vi "Taskbar Cleanup.vi"(4 "error in (no error)":errorcluster, 5 "hIcon":i32, 6 "hWnd":T1, 7 "siwutil32":T2) -> (0 "error out":errorcluster)   [LabVIEW 2011]
uses:
  Summitek EXT/Win32/SIWUTIL32/siwutil32.ctl
  Summitek EXT/Win32/WinUSER/Windows/hWnd.ctl
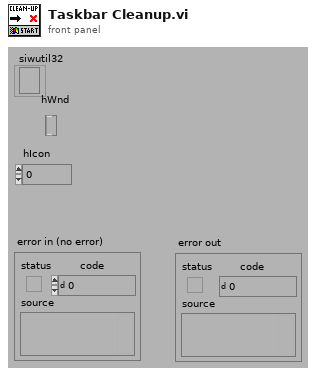
[diagram p1: front panel]
types:
  T1 = typedef "hWnd.ctl" = refnum<k1>
  T2 = typedef "siwutil32.ctl" = refnum<k7>
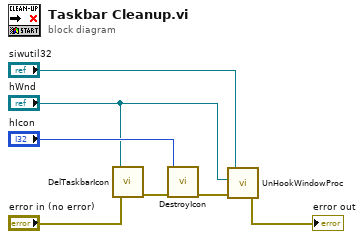
[diagram p0: block diagram]
diagram:
  n1 = call "DelTaskbarIcon.vi"("error in (no error)"="error in (no error)", "hWnd (NULL)"="hWnd") -> ("error out"=w3:errorcluster)  [unwired: 1 in, 4 out]
  n2 = call "DestroyIcon.vi"("error in (no error)"=w3, "hIcon"="hIcon") -> ("error out"=w2:errorcluster)  [unwired: 5 out]
  n3 = call "UnHookWindowProc.vi"("error in (no error)"=w2, "hWnd"="hWnd", "siwutil32"="siwutil32") -> ("error out"=→"error out":errorcluster)  [unwired: 4 out]
